vi "Get AlarmCode.vi"(8 "error in (no error)":errorcluster, 11 "Para":cluster{"url":string, "AccessToken":string}={"url"="http://data.watersystem.com.cn:50040", "AccessToken"="equip&GbbVkGRBUSaIfhTSjiolTAP8QMM"}) -> (0 "error out":errorcluster, 3 "project":T1)   [LabVIEW 2022 SP3, in "opSignIn.lvlib"]
uses:
  opSignIn.lvlib
  <vilib>/httpClient/POSTBuffer.vi
  <vilib>/httpClient/LabVIEWHTTPClient.lvlib
panel:
  out "body":string caption="体部"
  out "headers":string caption="头部"
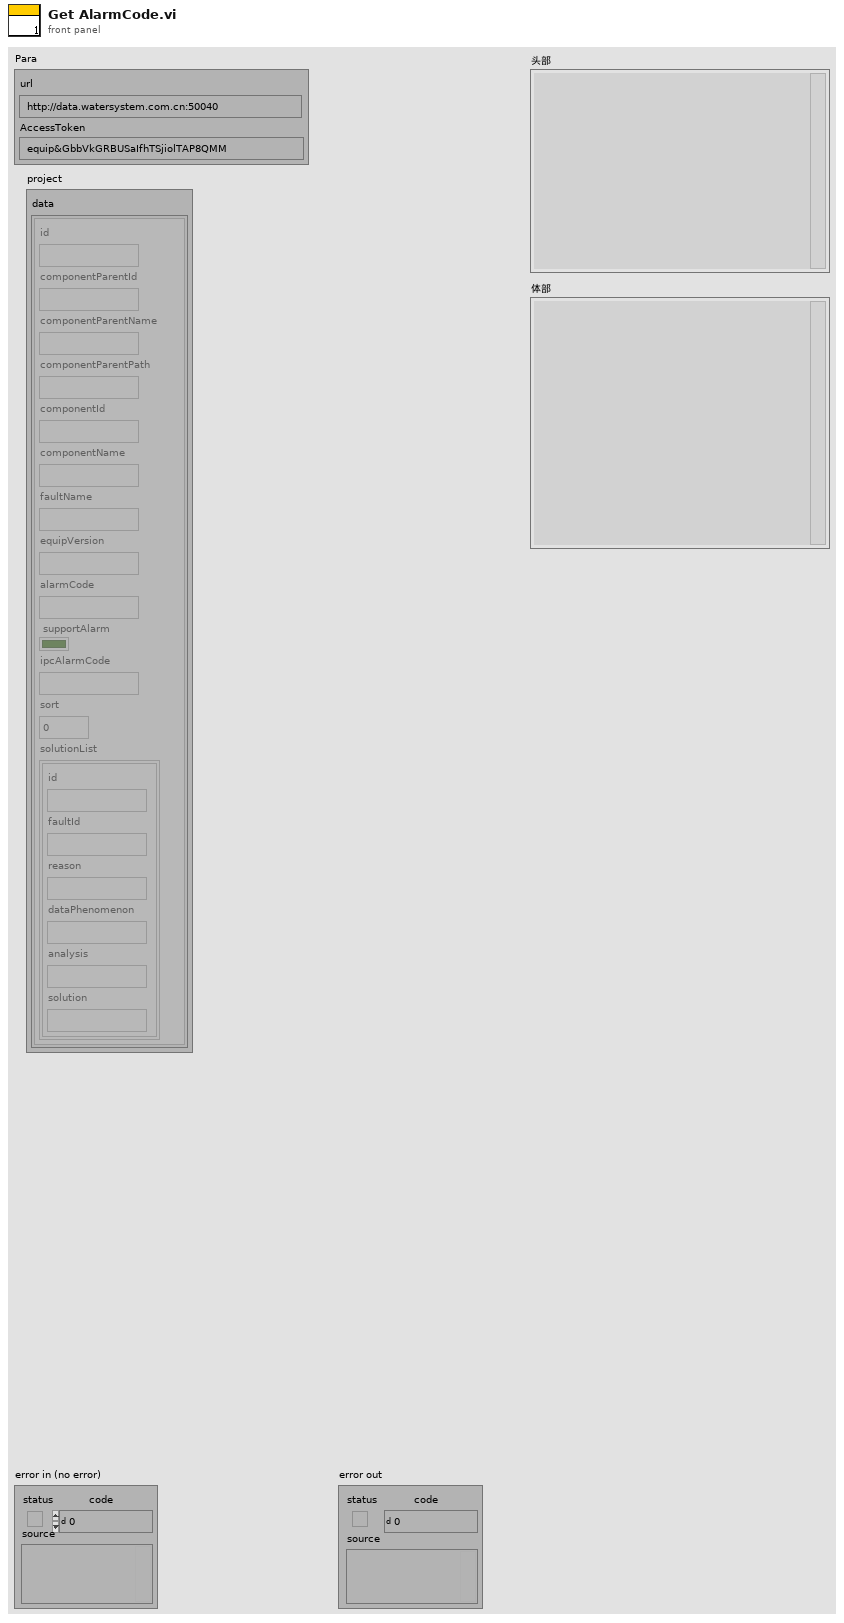
[diagram p1: front panel]
types:
  T1 = typedef "opSignIn.lvlib/报警格式.ctl" = cluster{"data":T2[]}
  T2 = typedef "opSignIn.lvlib/元素.ctl" = cluster{"id":string, "componentParentId":string, "componentParentName":string, "componentParentPath":string, "componentId":string, "componentName":string, "faultName":string, "equipVersion":string, "alarmCode":string, "supportAlarm":bool, "ipcAlarmCode":string, "sort":dbl, "solutionList":cluster{"id":string, "faultId":string, "reason":string, "dataPhenomenon":string, "analysis":string, "solution":string}[]}
  T3 = cluster{"code":string, "message":string, "success":bool}
  T4 = typedef "LabVIEWHTTPClient.lvlib/ClientHandle.ctl" = refnum<k1>
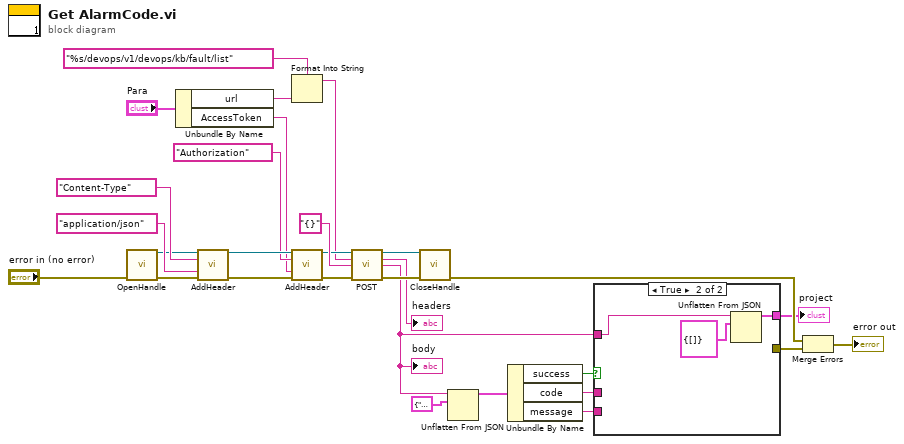
[diagram p0: block diagram]
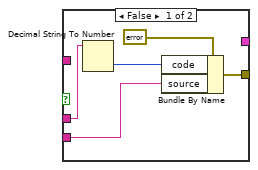
[diagram p2: hidden frame]
diagram:
  n1 = call <vilib>:"OpenHandle.vi"("error in (no error)"="error in (no error)") -> ("client handle out"=w24:T4, "error out"=w29:errorcluster)  [unwired: 13 in]
  n2 = Unbundle By Name("Para") -> ("url"=w13:string, "AccessToken"=w15:string)
  n3 = call <vilib>:"AddHeader.vi"("client handle"=w24, "header"="Content-Type", "value"="application/json", "error in (no error)"=w29) -> ("client handle out"=w25:T4, "error out"=w28:errorcluster)  [unwired: 10 in]
  n4 = Format Into String(format string="%s/devops/v1/devops/kb/fault/list" ("url"), w13) -> (resulting string=w14:string)  [unwired: 2 in, 1 out]
  n5 = call <vilib>:"AddHeader.vi"("client handle"=w25, "header"="Authorization", "value"=w15, "error in (no error)"=w28) -> ("client handle out"=w18:T4, "error out"=w19:errorcluster)  [unwired: 10 in]
  n6 = call-poly <vilib>:"POST.vi"("client handle"=w18, "url"=w14, "buffer"="{}", "error in (no error)"=w19) -> ("client handle out"=w17:T4, "headers"=→"headers":string, "body"=w1:string, "error out"=w23:errorcluster)  [unwired: 8 in]
  "body" <- w1
  n7 = call <vilib>:"CloseHandle.vi"("client handle"=w17, "error in (no error)"=w23) -> ("error out"=w6:errorcluster)  [unwired: 13 in]
  n8 = Unflatten From JSON(JSON string=w1, type and defaults=T3 {"code"="", "message"="", "success"=FALSE} ("response 2")) -> (value=w10:T3)  [unwired: 5 in, 1 out]
  n9 = Unbundle By Name(w10) -> ("success"=w9:bool, "code"=w8:string, "message"=w7:string)
  n10 = case shown="True" w9 {
    tunnel: w7 -> [w33 _]
    tunnel: [w32 _] -> w5
    tunnel: w8 -> [w31 _]
    tunnel: w1 -> [_ w36]
    tunnel: [_ w35] -> w3
    frame False {
      n11 = Decimal String To Number(string=w31) -> (number=w30:i32)  [unwired: 2 in, 1 out]
      n12 = Bundle By Name(cluster=errorcluster {"status"=TRUE, "code"=0, "source"=""} ("错误常量"), "code"=w30, "source"=w33) -> (w32:errorcluster)
    }
    frame True {
      n13 = Unflatten From JSON(JSON string=w36, type and defaults=T1 {"data"=[]} ("project")) -> (value=w35:T1)  [unwired: 5 in, 1 out]
    }
  }
  "project" <- w3
  n14 = Merge Errors(w6, w5) -> (→"error out":errorcluster)
